vi "Check Backpressure FIFO Space.vi"(6 "Read Success":bool, 8 "error in (no error)":errorcluster, 9 "Read Pos (from BP)":u32, 10 "Elements":u32, 11 "Write Pos":u32) -> (3 "Full":bool)   [LabVIEW 2021, in "CIF_NI_CIPC.lvlib"]
doc: "Check if there is remaining room in the FIFO for the writer by comparing the new write position to the last read position and the number of elements in the FIFO. This VI also needs to handle position rollover. The position rollover value changes based on the CIPC FIFO configuration so this needs to detect roll-over and latch the value. It then needs to adjust for roll-over in the write position until the read position has also rolled over. \n\nNote, this retains history so only one instance can be called per FIFO."
uses:
  CIF_NI_CIPC.lvlib
  <vilib>/CIF Foundation/CIF Utilities/Boolean/Boolean_CIF_U.lvlib
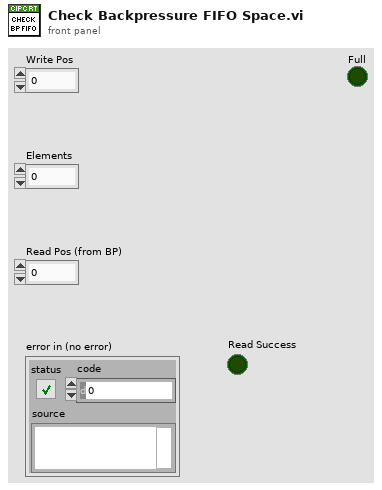
[diagram p1: front panel]
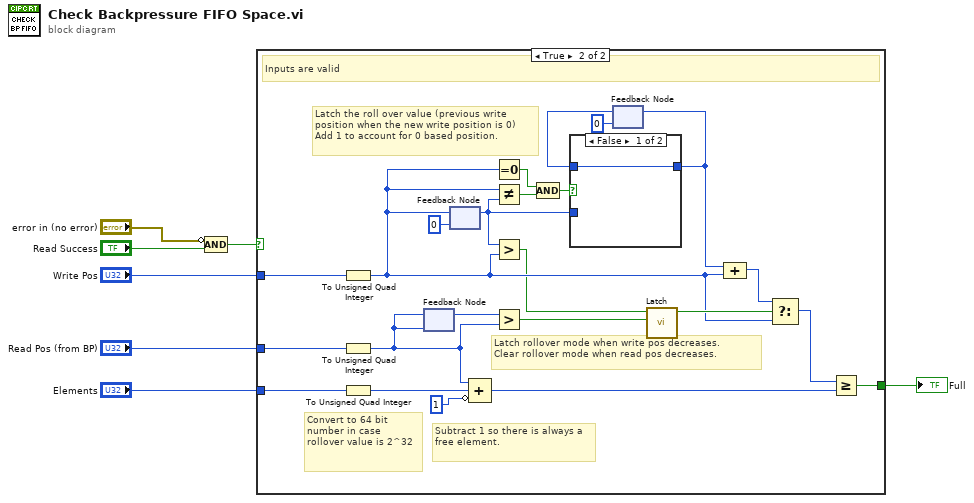
[diagram p0: block diagram]
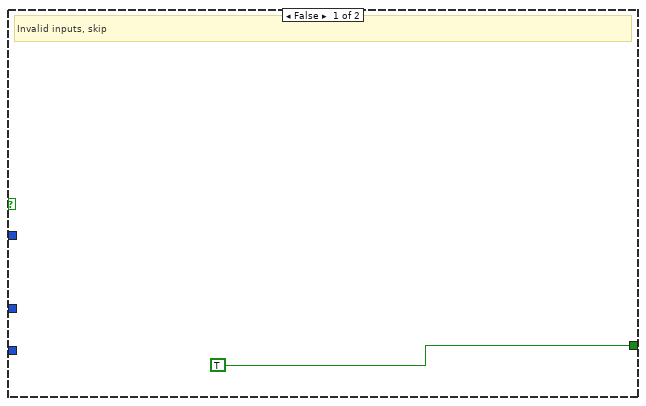
[diagram p2: hidden frame]
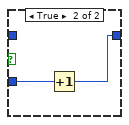
[diagram p3: hidden frame]
diagram:
  n1 = Compound Arithmetic op=AND(invert "error in (no error)", "Read Success") -> (w1:bool)
  n2 = case shown="True" w1 {
    tunnel: "Write Pos" -> [_ w29]
    tunnel: "Read Pos (from BP)" -> [_ w27]
    tunnel: [TRUE w25] -> w5
    tunnel: "Elements" -> [_ w18]
    frame False {
      # "Invalid inputs, skip"
    }
    frame True {
      # "Subtract 1 so there is always a free element."
      # "Convert to 64 bit number in case rollover value is 2^32"
      # "Latch rollover mode when write pos decreases.\nClear rollover mode when read pos decreases."
      # "Latch the roll over value (previous write position when the new write position is 0) Add 1 to account for 0 based position."
      # "Inputs are valid"
      n3 = To Unsigned Quad Integer(1:w29) -> (0:w11:u64)
      n4 = To Unsigned Quad Integer(1:w27) -> (0:w14:u64)
      n5 = To Unsigned Quad Integer(1:w18) -> (0:w26:u64)
      n6 = feedback #1(w14) -> (w15:u64)
      n7 = feedback-in #1(w14) -> ()
      n8 = feedback #2(u64 0 ("Write Pos")) -> (w12:u64)
      n9 = feedback-in #2(w11) -> ()
      n10 = Compound Arithmetic op=ADD(w14, w26, invert u64 1 ("value")) -> (w24:u64)
      n11 = Equal To 0?(x=w11) -> (x = 0?=w9:bool)
      n12 = Not Equal?(x=w11, y=w12) -> (x != y?=w31:bool)
      n13 = Greater?(x=w12, y=w11) -> (0:w10:bool)
      n14 = Greater?(x=w15, y=w14) -> (0:w13:bool)
      n15 = Compound Arithmetic op=AND(w9, w31) -> (w23:bool)
      n16 = feedback #3(u64 0) -> (w22:u64)
      n17 = case shown="False" w23 {
        tunnel: w12 -> [_ w34]
        tunnel: [w32 w33] -> w20
        tunnel: w22 -> [w32 _]
        frame False {
        }
        frame True {
          n18 = Increment(x=w34) -> (x+1=w33:u64)
        }
      }
      n19 = feedback-in #3(w20) -> ()
      n20 = call <vilib>:"Latch.vi"("clear"=w13, "set"=w10) -> ("out"=w17:bool)  [unwired: 9 in]
      n21 = Compound Arithmetic op=ADD(w20, w11) -> (w28:u64)
      n22 = Select(t=w28, s=w17, f=w11) -> (s? t:f=w19:u64)
      n23 = Greater Or Equal?(x=w19, y=w24) -> (x >= y?=w25:bool)
    }
  }
  "Full" <- w5
